vi "Signal acquisition on external trigger.vi"() -> ()   [LabVIEW 2010]
doc: "This example shows how to acquire 16k samples of signal on fast analog inputs. Signal will be acquired when the external trigger condition is meet. Time length of the acquired signal depends on the time scale of a buffer that can be set with a decimation factor. Decimations and time scales of a buffer are given in the table below. Voltage range of fast analog inputs on the Red Pitaya depends on gain setting that can be set by jumpers. HV setting is for input range to ±20V, while LV sets input range to ±1V."
uses:
  RedPitaya.lvlib
panel:
  in  "Trigger Level (0 mV)":i32=100
  in  "Delay (# Samples)":i32 max=16348
  in  "Decimation":u32(ring)=8 items=["65536"=65536, "8192"=8192, "1024"=1024, "64"=64, "8"=8, "1"=1]
  in  "IP address":string="192.168.1.100"
  out "Waveform Graph":dbl[](graph)
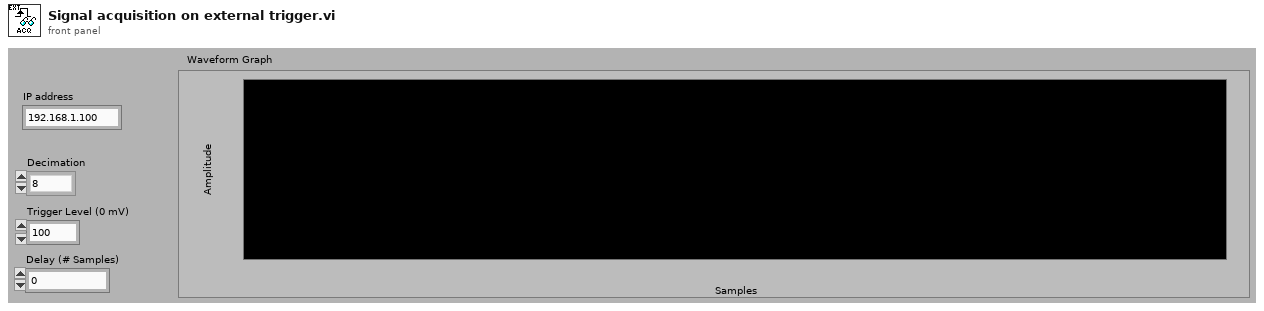
[diagram p1: front panel]
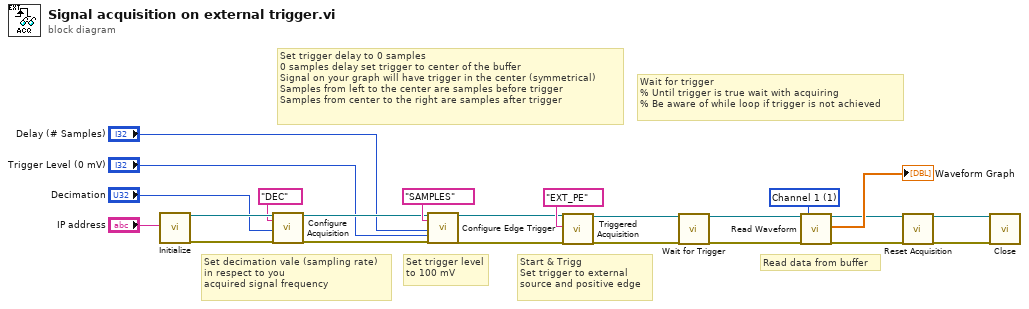
[diagram p0: block diagram]
diagram:
  w22 = u16 1 items=["Channel 1"=1, "Channel 2"=2] ("Channel (1|2)")
  # "Read data from buffer"
  # "Start & Trigg\nSet trigger to external\nsource and positive edge"
  # "Wait for trigger\n% Until trigger is true wait with acquiring\n% Be aware of while loop if trigger is not achieved"
  # "Set trigger delay to 0 samples\n0 samples delay set trigger to center of the buffer\nSignal on your graph will have trigger in the center (symmetrical)\nSamples from left to the center are samples before trigger \nSamples from center to the right are samples after trigger"
  # "Set trigger level\nto 100 mV"
  # "Set decimation vale (sampling rate)\nin respect to you \nacquired signal frequency"
  n1 = call "Initialize.vi"("IP address"="IP address") -> ("RedPitaya TCP Connection"=w7:refnum<k5>, "error out"=w6:errorcluster)  [unwired: 17 in]
  n2 = call "Configure Acquisition.vi"("RedPitaya connection in"=w7, "Decimation/Sampling Rate"="DEC", "Decimation"="Decimation", "error in"=w6) -> ("RedPitaya connection out"=w8:refnum<k5>, "error out"=w4:errorcluster)  [unwired: 14 in]
  n3 = call "Configure Edge Trigger.vi"("RedPitaya connection in"=w8, "Trigger Delay mode"="SAMPLES", "Delay (# Samples)"="Delay (# Samples)", "Trigger Level (0 mV)"="Trigger Level (0 mV)", "error in"=w4) -> ("RedPitaya connection out"=w20:refnum<k5>, "error out"=w19:errorcluster)  [unwired: 13 in]
  n4 = call "Triggered Acquisition.vi"("RedPitaya TCP connection in"=w20, "Trigger Mode"="EXT_PE", "error in"=w19) -> ("RedPitaya TCP connection out"=w16:refnum<k5>, "error out"=w13:errorcluster)  [unwired: 15 in]
  n5 = call "Wait for Trigger.vi"("RedPitaya TCP connection in"=w16, "error in"=w13) -> ("RedPitaya TCP connection out"=w15:refnum<k5>, "error out"=w14:errorcluster)  [unwired: 16 in]
  n6 = call "Read Waveform.vi"("RedPitaya TCP Connection in"=w15, "error in"=w14, "Channel #"=w22) -> ("RedPitaya TCP Connection out"=w12:refnum<k5>, "Measurement Array"=→"Waveform Graph":dbl[], "error out"=w10:errorcluster)  [unwired: 14 in]
  n7 = call "Reset Acquisition.vi"("RedPitaya connection in"=w12, "error in"=w10) -> ("RedPitaya connection out"=w11:refnum<k5>, "error out"=w9:errorcluster)  [unwired: 16 in]
  n8 = call "Close.vi"("connection ID"=w11, "error in"=w9) -> ()  [unwired: 17 in, 1 out]
